vi "ReferencedVariables_CreateReferenceVariable_6x8x6.vi"(0 "reference in":refnum<class>, 2 "InitalValue":T1, 5 "error in (no error)":errorcluster) -> (14 "reference out":refnum<class>, 16 "ReferenceVariableOut":refnum<data-value>, 19 "error out":errorcluster)   [LabVIEW 2020]
doc: "This VI creates a DVR reference for a variable."
uses:
  <resource>/Framework/Providers/Open_GDS/ClassProviders/DesignPatterns/ReferencedVariables/ReferencedVariables_SubVIs/ReferencedVariable.ctl
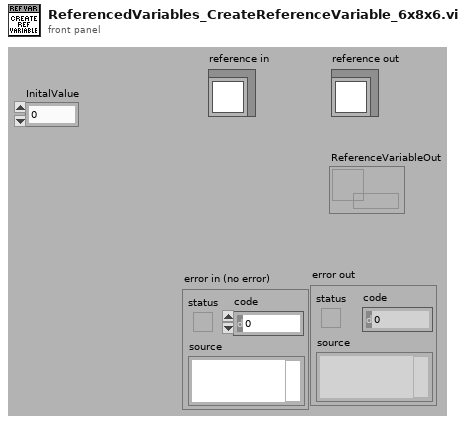
[diagram p1: front panel]
types:
  T1 = typedef "ReferencedVariable.ctl" = i32
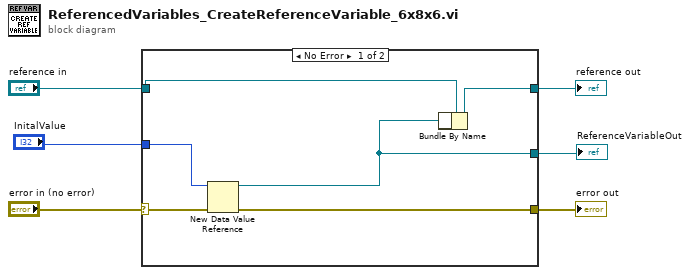
[diagram p0: block diagram]
diagram:
  n1 = case shown="No Error" "error in (no error)" {
    selector: "error in (no error)" -> [w12 w13]
    tunnel: [w9 w14] -> w6
    tunnel: [w11 w13] -> w5
    tunnel: "reference in" -> [w10 w14]
    tunnel: "InitalValue" -> [w7 _]
    tunnel: [w8 _] -> w2
    frame No Error {
      n2 = New Data Value Reference(data value=w7, error in=w12) -> (data value reference=w8:refnum<data-value>, error out=w11:errorcluster)
      n3 = Bundle By Name(cluster=w10, w8) -> (w9:refnum<class>)
    }
    frame Error {
    }
  }
  "error out" <- w5
  "reference out" <- w6
  "ReferenceVariableOut" <- w2
